vi "MAIN AVERAGE CHECK.vi"() -> ()   [LabVIEW 2018]
uses:
  <vilib>/FPGAPlugInAG/cRIO-9082/niLvFpga_Open_cRIO-9082.vi
  <vilib>/rvi/interface/common/dynamic/niFpgaDynamicAddResources.vi
  <vilib>/FPGAPlugInAG/Dynamic/niLvFpga_Reset_Dynamic.vi
  <vilib>/FPGAPlugInAG/Dynamic/niLvFpga_Run_Dynamic.vi
  <vilib>/Utility/error.llb/Error Cluster From Error Code.vi
  <vilib>/rvi/errors/niLvFpgaAdjustHostInterfaceError.vi
  <vilib>/FPGAPlugInAG/Dynamic/niLvFpga_Abort_Dynamic.vi
  <vilib>/FPGAPlugInAG/Dynamic/niLvFpga_Close_Dynamic.vi
  <vilib>/rvi/interface/nirviOpenFPGA/nirviOpenFPGA.xnode
  FPGA Bitfiles/25032021 FPGA main.lvbitx
  <vilib>/rvi/interface/nirviMethod/nirviMethod.xnode
  <vilib>/rvi/interface/nirviReadWriteControl/nirviReadWriteControl.xnode
  <vilib>/rvi/interface/nirviCloseFPGA/nirviCloseFPGA.xnode
  <vilib>/ptbypt/NI_PtbyPt.lvlib
  NiFpgaLv.dll
  <vilib>/rvi/interface/Simulation/niFpgaSimulationCallBeginRW.vi
panel:
  out "Mean Data":dbl[](array[numeric])
  out "Numeric":u32
  out "Numeric 2":i32
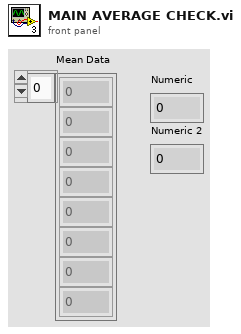
[diagram p1: front panel]
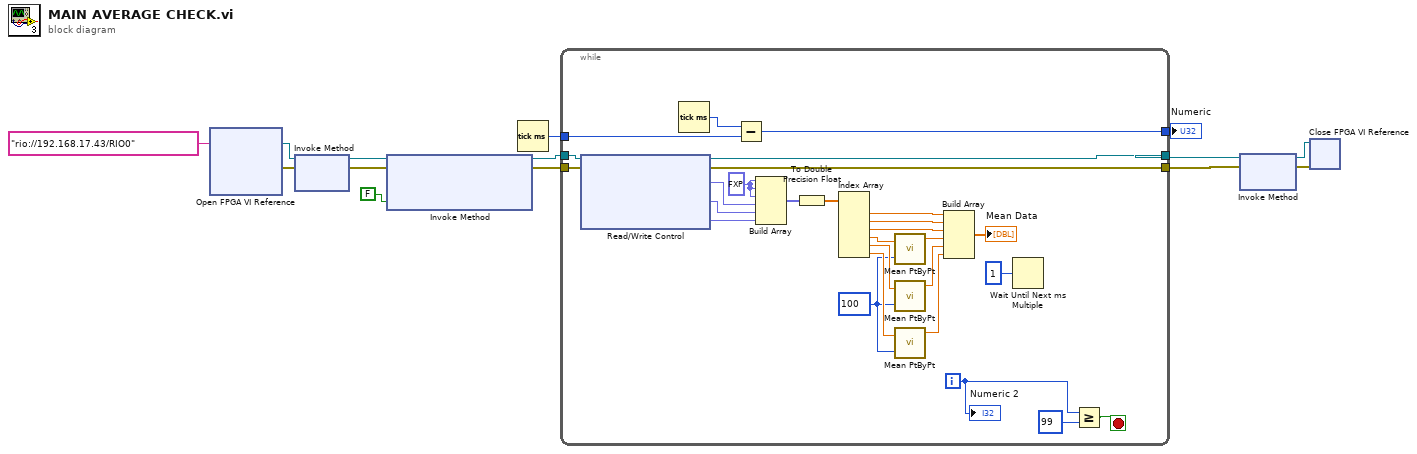
[diagram p0: block diagram]
diagram:
  n1 = xnode "Open FPGA VI Reference"("resource name"=tag "rio://192.168.17.43/RIO0") -> ("FPGA VI Reference Out"=w10:refnum<k20>, "error out"=w11:errorcluster)  [unwired: 1 in]
  n2 = xnode "Invoke Method"("FPGA VI Reference In"=w10, "error in"=w11) -> ("FPGA VI Reference Out"=w12:refnum<k20>, "error out"=w13:errorcluster)
  n3 = xnode "Invoke Method"("FPGA VI Reference In"=w12, "error in"=w13, "Wait Until Done (F)"=FALSE) -> ("FPGA VI Reference Out"=w7:refnum<k20>, "error out"=w6:errorcluster)
  n4 = Tick Count (ms)() -> (millisecond timer value=w14:u32)
  n5 = while {
    tunnel: [w37] -> w3
    tunnel: w14 -> [w32]
    tunnel: w7 -> [w36]
    tunnel: w6 -> [w35]
    tunnel: [w34] -> w2
    tunnel: [w31] -> w1
    i -> [w17]
    stop <- w15 stop-if-true
    w18 = fxp<+/-,24,5> 0.0 ("element")
    w20 = 100 ("sample length")
    n6 = xnode "Read/Write Control"("FPGA VI Reference In"=w36, "error in"=w35) -> ("FPGA VI Reference Out"=w37:refnum<k20>, "error out"=w34:errorcluster, "Mod8/Torque  L"=w39:fxp<+/-,24,5>, "Mod8/Torque  R"=w40:fxp<+/-,24,5>, "Mod8/Torque  H"=w41:fxp<+/-,24,5>)
    n7 = Tick Count (ms)() -> (millisecond timer value=w33:u32)
    n8 = Subtract(x=w33, y=w32) -> (x-y=w31:u32)
    n9 = Build Array(w18, w18, w18, w39, w40, w41) -> (w42:fxp<+/-,24,5>[])
    n10 = To Double Precision Float(number=w42) -> (double precision float=w19:dbl[])
    n11 = Index Array(array=w19) -> (element #1=w25:dbl, element #2=w24:dbl, element #3=w23:dbl, element #4=w30:dbl, element #5=w29:dbl, element #6=w22:dbl)  [unwired: 6 in]
    n12 = call <vilib>:"Mean PtByPt.vi"("x"=w30, "sample length"=w20) -> ("mean"=w28:dbl)  [unwired: 2 in, 1 out]
    n13 = call <vilib>:"Mean PtByPt.vi"("x"=w29, "sample length"=w20) -> ("mean"=w27:dbl)  [unwired: 2 in, 1 out]
    n14 = call <vilib>:"Mean PtByPt.vi"("x"=w22, "sample length"=w20) -> ("mean"=w21:dbl)  [unwired: 2 in, 1 out]
    n15 = Build Array(w25, w24, w23, w28, w27, w21) -> (→"Mean Data":dbl[])
    n16 = Wait Until Next ms Multiple(millisecond multiple=u32 1) -> ()  [unwired: 1 out]
    n17 = Greater Or Equal?(x=w17, y=99) -> (x >= y?=w15:bool)
    "Numeric 2" <- w17
  }
  "Numeric" <- w1
  n18 = xnode "Invoke Method"("FPGA VI Reference In"=w3, "error in"=w2) -> ("FPGA VI Reference Out"=w5:refnum<k20>, "error out"=w4:errorcluster)
  n19 = xnode "Close FPGA VI Reference"("FPGA VI Reference In"=w5, "error in"=w4) -> ()  [unwired: 1 out]
